vi "chart series set labels custom.vi"(8 "error in (no error)":errorcluster, 10 "data_labels":u32, 11 "series":u32) -> (0 "error out":errorcluster, 3 "function return":u32(ring))   [LabVIEW 8.6]
doc: "lxw_error chart_series_set_labels_custom(lxw_chart_series series, unsigned long data_labels);"
uses:
  pending_lvxlsxwriter/xlsxwriter.dll
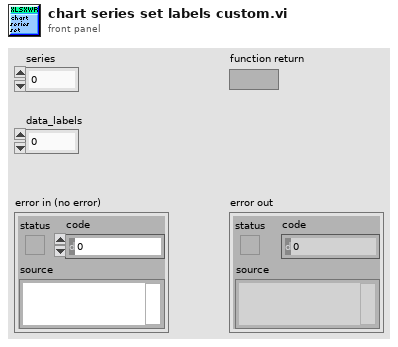
[diagram p1: front panel]
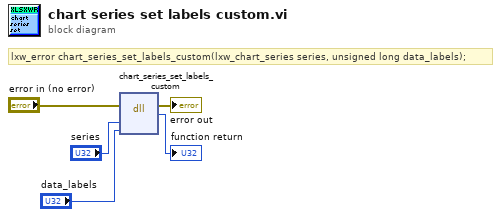
[diagram p0: block diagram]
diagram:
  # "lxw_error chart_series_set_labels_custom(lxw_chart_series series, unsigned long data_labels);"
  n1 = dll-call lib="C:/Users/WDAGUtilityAccount/Desktop/pending_lvxlsxwriter/xlsxwriter.*" fn="chart_series_set_labels_custom"(error in="error in (no error)", "series"="series", "data_labels"="data_labels") -> (error out=→"error out":errorcluster, →"function return":u32)  [unwired: 4 in, 1 out]
